vi "LaunchAppender.vi"(8 "error in (no error)":errorcluster, 10 "Lumberjack.lvlib:Appender.lvclass":refnum<class "Appender.lvclass">, 11 "LogManager in":refnum<class "LogManager.lvclass">) -> (0 "error out":errorcluster, 3 "LogManager out":refnum<class "LogManager.lvclass">)   [LabVIEW 2026, in "Lumberjack.lvlib" / "LogManager.lvclass"]
doc: "Launch a constructed, configured Appender as a nested actor of the LogManager and register it. Reads the appender's id via GetID and checks the registry for a duplicate: if the id is already present, the appender is ignored gracefully with a warning (LumberjackErrorBase + 27, status FALSE) and is neither launched nor added, so ids remain unique and id-based operations (unregister, configure) stay unambiguous. Otherwise the appender is launched with Launch Nested Actor (tying its lifecycle to the manager, so stopping the manager stops it), and a {id, enqueuer} entry is added to the registry. Does not post the Snapshot; the caller invokes PostSnapshot afterward. Called by Actor Core for the default file appender and by RegisterAppenderMsg for additional appenders (SRS-LMBR-045)."
uses:
  LogManager.lvclass
  Appenders/Appender.lvclass/Appender.lvclass
  LogManager.lvclass/LogManager.ctl
  TypeDefs/RegistryEntry.ctl
  <vilib>/ActorFramework/Message Enqueuer/Message Enqueuer.lvclass
  Lumberjack.lvlib
  <vilib>/ActorFramework/Actor/Actor.lvclass
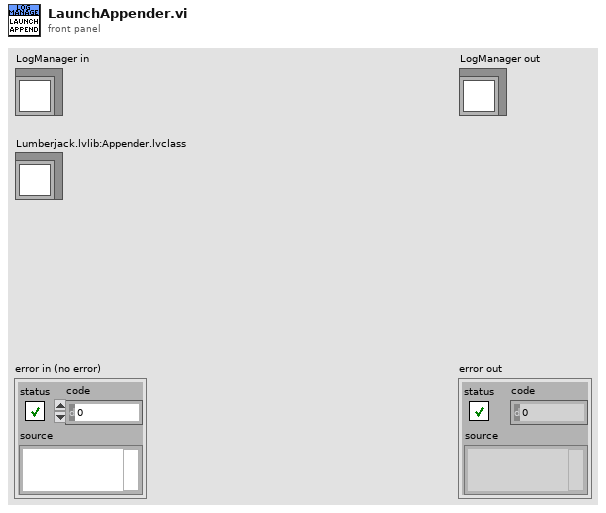
[diagram p1: front panel]
types:
  T1 = typedef "Lumberjack.lvlib/RegistryEntry.ctl" = cluster{"id":string, "enqueuer":refnum<class "Message Enqueuer.lvclass">}
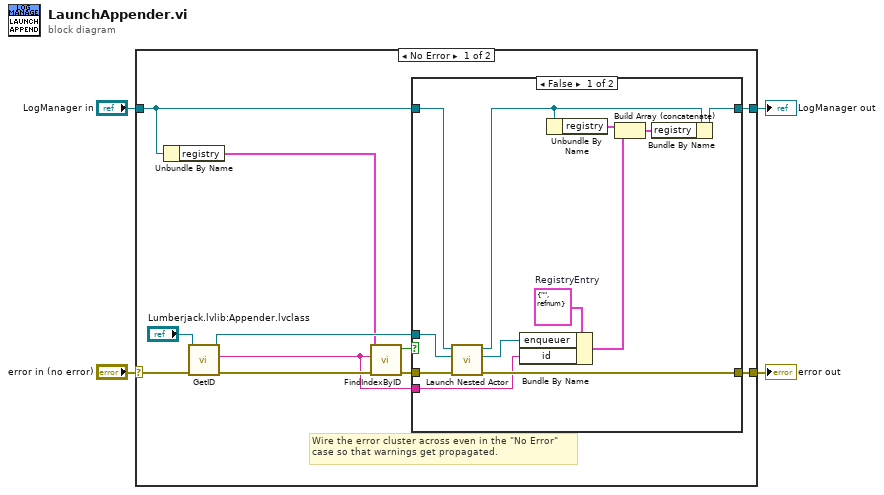
[diagram p0: block diagram]
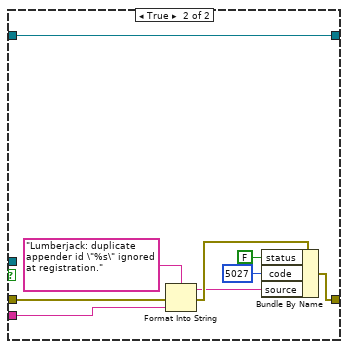
[diagram p2: hidden frame]
diagram:
  n1 = case shown="No Error" "error in (no error)" {
    selector: "error in (no error)" -> [w14 w38]
    tunnel: [w12 w38] -> w3
    tunnel: [w11 w37] -> w1
    tunnel: "LogManager in" -> [w10 w37]
    frame No Error {
      # "Wire the error cluster across even in the \"No Error\"\ncase so that warnings get propagated."
      n2 = Unbundle By Name(w10) -> ("registry"=w7:T1[])
      n3 = call "GetID.vi"("error in (no error)"=w14, "Appender in"="Lumberjack.lvlib:Appender.lvclass") -> ("error out"=w9:errorcluster, "ID"=w5:string, "Appender out"=w13:refnum<class "Appender.lvclass">)  [unwired: 7 in]
      n4 = call "FindIndexByID.vi"("error in (no error)"=w9, "id"=w5, "registry"=w7) -> ("error out"=w8:errorcluster, "found"=w6:bool)  [unwired: 5 in, 2 out]
      n5 = case shown="False" w6 {
        tunnel: w13 -> [w26 _]
        tunnel: w8 -> [w24 w30]
        tunnel: [w23 w29] -> w12
        tunnel: [w22 w36] -> w11
        tunnel: w10 -> [w18 w36]
        tunnel: w5 -> [w17 w28]
        frame False {
          w27 = T1 {"id"="", "enqueuer"=refnum}  # RegistryEntry
          n6 = call <vilib>:"Launch Nested Actor.vi"("error in (no error)"=w24, "Nested Actor"=w26, "Caller Actor in"=w18) -> ("error out"=w23:errorcluster, "Nested Actor's Enqueuer"=w25:refnum<class "Message Enqueuer.lvclass">, "Caller Actor out"=w16:refnum<class "LogManager.lvclass">)  [unwired: 6 in]
          n7 = Bundle By Name(cluster=w27, "enqueuer"=w25, "id"=w17) -> (w20:T1)
          n8 = Unbundle By Name(w16) -> ("registry"=w21:T1[])
          n9 = Build Array (concatenate)(w21, w20) -> (w19:T1[])
          n10 = Bundle By Name(cluster=w16, "registry"=w19) -> (w22:refnum<class "LogManager.lvclass">)
        }
        frame True {
          n11 = Format Into String(format string="Lumberjack: duplicate appender id \"%s\" ignored at registration." ("source"), error in=w30, w28) -> (resulting string=w34:string, error out=w35:errorcluster)  [unwired: 1 in]
          n12 = Bundle By Name(cluster=w35, "status"=FALSE, "code"=5027, "source"=w34) -> (w29:errorcluster)
        }
      }
    }
    frame Error {
    }
  }
  "error out" <- w3
  "LogManager out" <- w1
